vi "Write Group Name.vi"(8 "error in (no error)":errorcluster, 10 "Group Name":string, 11 "Logging Data in":refnum<class "Logging Data.lvclass">) -> (0 "error out":errorcluster, 3 "Logging Data out":refnum<class "Logging Data.lvclass">)   [LabVIEW 2024, in "Logging Data.lvlib" / "Logging Data.lvclass"]
uses:
  Logging Data.lvclass
  Logging Data.lvclass/Logging Data.ctl
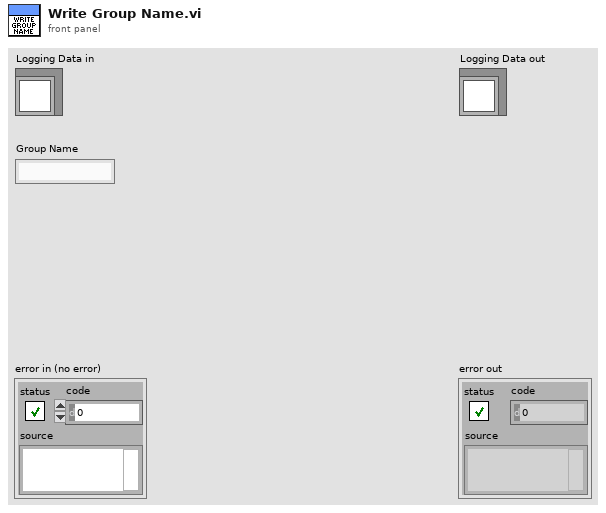
[diagram p1: front panel]
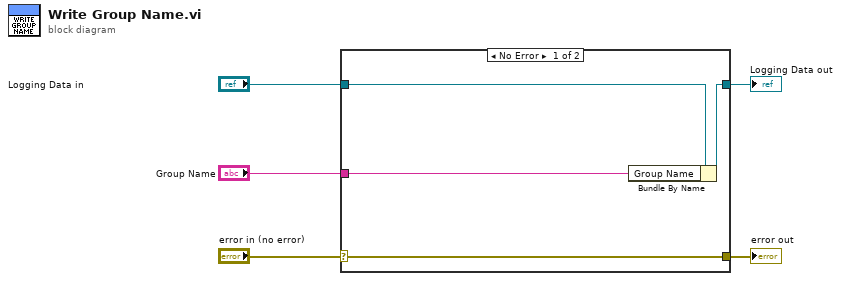
[diagram p0: block diagram]
diagram:
  n1 = case shown="No Error" "error in (no error)" {
    selector: "error in (no error)" -> [w9 w10]
    tunnel: [w9 w10] -> w4
    tunnel: [w7 w11] -> w2
    tunnel: "Logging Data in" -> [w8 w11]
    tunnel: "Group Name" -> [w6 _]
    frame No Error {
      n2 = Bundle By Name(cluster=w8, "Group Name"=w6) -> (w7:refnum<class "Logging Data.lvclass">)
    }
    frame Error {
    }
  }
  "error out" <- w4
  "Logging Data out" <- w2
